vi "test Get Multiple Tables as JSON.vi"(11 "Test Case In":refnum<class "Test Config From Excel Table.lvclass">) -> (0 "error out":errorcluster, 3 "Test Case Out":refnum<class "Test Config From Excel Table.lvclass">)   [LabVIEW 2020, in "Test Config From Excel Table.lvclass"]
uses:
  Test Config From Excel Table.lvclass
  C:/Program Files/National Instruments/LabVIEW 2025/vi.lib/Astemes/LUnit/Test Case.lvclass
  Source/Config from Excel Table/Config from Excel Table.lvclass
  <vilib>/Astemes/LUnit/Test Case.lvclass/Test Case.ctl
  <vilib>/JDP Science/JSONtext/JSONtext.lvlib
  <vilib>/Astemes/LUnit/Test Case.lvclass
  Open-Xml-LabVIEW/Source/Open Xml.lvlib
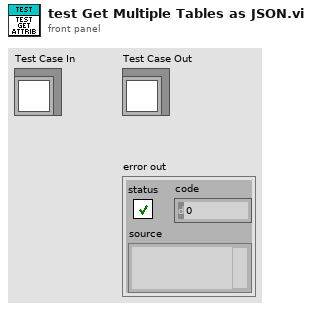
[diagram p1: front panel]
types:
  T1 = cluster{"Sheet Name":string, "Name":string, "Display Name":string, "Range or Cell Address":string}
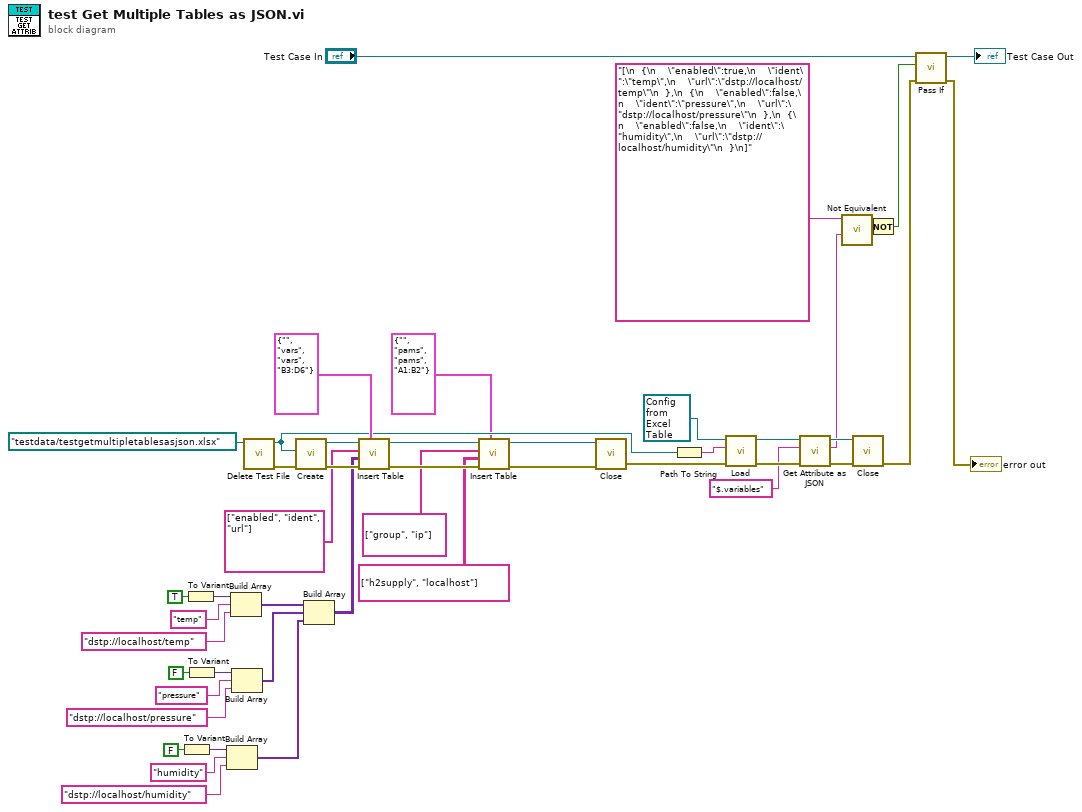
[diagram p0: block diagram]
diagram:
  n1 = To Variant(anything=FALSE) -> (Variant=w19:variant)
  n2 = To Variant(anything=TRUE) -> (Variant=w28:variant)
  n3 = To Variant(anything=FALSE) -> (Variant=w22:variant)
  n4 = Build Array(w19, "humidity", "dstp://localhost/humidity") -> (w15:variant[])
  n5 = Build Array(w28, "temp", "dstp://localhost/temp") -> (w25:variant[])
  n6 = Build Array(w22, "pressure", "dstp://localhost/pressure") -> (w16:variant[])
  n7 = call "Delete Test File.vi"("name or relative path"=path "testdata/testgetmultipletablesasjson.xlsx") -> ("error out"=w33:errorcluster, "deleted path"=w7:path)  [unwired: 9 in]
  n8 = call "Create.vi"("error in"=w33, "Path"=w7) -> ("error out"=w32:errorcluster, "SpreadsheetDoc"=w13:refnum<k24>)  [unwired: 8 in]
  n9 = Build Array(w25, w16, w15) -> (w14:variant[][])
  n10 = call "Insert Table.vi"("Location"=T1 {"Sheet Name"="", "Name"="vars", "Display Name"="vars", "Range or Cell Address"="B3:D6"}, "error in"=w32, "Cell Values"=w14, "Header Names"=string[] ["enabled", "ident", "url"], "SpreadsheetDoc in"=w13) -> ("error out"=w12:errorcluster, "SpreadsheetDoc out"=w5:refnum<k24>)  [unwired: 5 in]
  n11 = call "Insert Table.vi"("Location"=T1 {"Sheet Name"="", "Name"="pams", "Display Name"="pams", "Range or Cell Address"="A1:B2"}, "error in"=w12, "Cell Values"=string[][] [["h2supply", "localhost"]], "Header Names"=string[] ["group", "ip"], "SpreadsheetDoc in"=w5) -> ("error out"=w6:errorcluster, "SpreadsheetDoc out"=w4:refnum<k24>)  [unwired: 5 in]
  n12 = call "Close.vi"("error in"=w6, "SpreadsheetDoc"=w4) -> ("error out"=w11:errorcluster)  [unwired: 9 in]
  n13 = Path To String(path=w7) -> (string=w43:string)
  n14 = call-dynamic "Load.vi"("error in"=w11, "Source"=w43, "Config from Excel Table in"=refnum<class "Config from Excel Table.lvclass"> refnum ("Config from EXCEL Table.lvclass")) -> ("error out"=w40:errorcluster, "Config from Excel Table out"=w41:refnum<class "Config from Excel Table.lvclass">)  [unwired: 7 in]
  n15 = call-dynamic "Get Attribute as JSON.vi"("error in"=w40, "Attribute"="$.variables", "Config from Excel Table in"=w41) -> ("error out"=w38:errorcluster, "<JSON>"=w34:string, "Config from Excel Table out"=w37:refnum<class "Config from Excel Table.lvclass">)  [unwired: 6 in]
  n16 = call <vilib>:"Not Equivalent.vi"("Other JSON"=w34, "JSON"="[\n  {\n    \"enabled\":true,\n    \"ident\":\"temp\",\n    \"url\":\"dstp://localhost/temp\"\n  },\n  {\n    \"enabled\":false,\n    \"ident\":\"pressure\",\n    \"url\":\"dstp://localhost/pressure\"\n  },\n  {\n    \"enabled\":false,\n    \"ident\":\"humidity\",\n    \"url\":\"dstp://localhost/humidity\"\n  }\n]" ("<JSON>")) -> ("Not Equivalent"=w36:bool)  [unwired: 8 in]
  n17 = call-dynamic "Close.vi"("error in"=w38, "Config from Excel Table in"=w37) -> ("error out"=w42:errorcluster)  [unwired: 8 in, 1 out]
  n18 = Not(x=w36) -> (.not. x?=w35:bool)
  n19 = call <vilib>:"Pass If.vi"("error in (no error)"=w42, "Pass?"=w35, "LUnit Test Case In"="Test Case In") -> ("error out"=→"error out":errorcluster, "LUnit Test Case Out"=→"Test Case Out":refnum<class "Test Config From Excel Table.lvclass">)  [unwired: 7 in]
